vi "Close Key.vi"(8 "error in (no error)":errorcluster, 11 "CngKey in":refnum<k24>) -> (0 "error out":errorcluster)   [LabVIEW 2021, in "dotNET Crypto Key Management.lvlib"]
doc: "Disposes and closes the reference to the key(s)."
uses:
  dotNET Crypto Key Management.lvlib
  System.Core
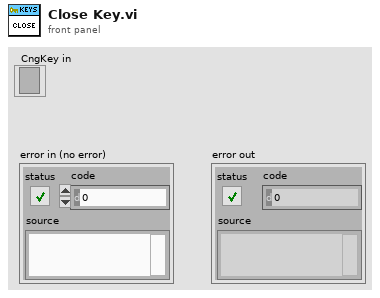
[diagram p1: front panel]
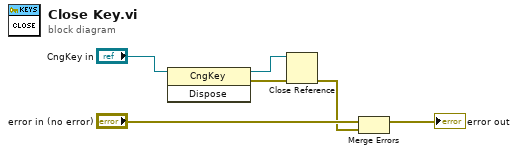
[diagram p0: block diagram]
diagram:
  n1 = invoke class="CngKey" method="Dispose"(reference="CngKey in") -> (reference out=w5:refnum<k24>, error out=w4:errorcluster)  [unwired: 2 in, 1 out]
  n2 = Close Reference(reference=w5, error in (no error)=w4) -> (error out=w1:errorcluster)
  n3 = Merge Errors("error in (no error)", w1) -> (→"error out":errorcluster)
